vi "Check Database Exists.vi"(8 "Error In":errorcluster) -> (0 "error out":errorcluster, 2 "Error Message":string, 3 "Database Error?":bool=TRUE)   [LabVIEW 2020]
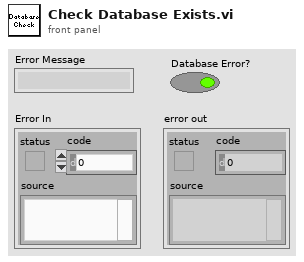
[diagram p1: front panel]
types:
  T1 = typedef "NI_Database_API.lvlib/Conn ObjectReference.ctl" = refnum<k1>
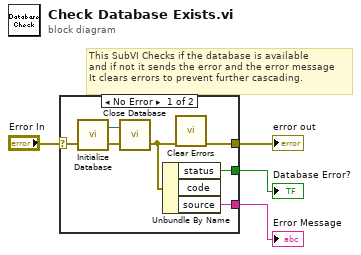
[diagram p0: block diagram]
diagram:
  # "This SubVI Checks if the database is available \nand if not it sends the error and the error message\nIt clears errors to prevent further cascading."
  n1 = case shown="No Error" "Error In" {
    selector: "Error In" -> [w9 w12]
    tunnel: [w8 w12] -> w3
    tunnel: [w6 _] -> w2
    tunnel: [w5 _] -> w1
    frame No Error {
      n2 = call "Initialize Database.vi"("Error In"=w9) -> ("Error Out"=w11:errorcluster, "Database Connection Out"=w10:T1)  [unwired: 1 in]
      n3 = call "Close Database.vi"("Error In"=w11, "Database Full Information In"=w10) -> ("Error Out"=w7:errorcluster)  [unwired: 1 in]
      n4 = Unbundle By Name(w7) -> ("status"=w6:bool, "source"=w5:string)  [unwired: 1 out]
      n5 = call <vilib>:"Clear Errors.vi"("error in (no error)"=w7) -> ("error out"=w8:errorcluster)  [unwired: 5 in, 1 out]
    }
    frame Error {
    }
  }
  "error out" <- w3
  "Database Error?" <- w2
  "Error Message" <- w1
